vi "test Encode and Decoding Parameters for Payload.vi"() -> ()   [LabVIEW 2020, in "AIM ARINC 664 Scripting.lvclass"]
uses:
  AIM ARINC 664 Scripting.lvclass
  Shared/Encoding (Arinc664).ctl
  <vilib>/addons/_JKI Toolkits/VI Tester/TestCase.llb/TestCase.lvclass
  Engine/Implementation/Rx UDP Execution Unit/Rx UDP Execution Unit.lvclass
  C:/Program Files (x86)/National Instruments/LabVIEW 2020/vi.lib/addons/_JKI Toolkits/VI Tester/TestCase.llb/TestCase.lvclass
panel:
  out "Message Buffer out":u8[](array[numeric])
  out "Data":u8[](array[numeric])
  out "Array":dbl[](array[numeric])
  out "TestCase out":refnum<class "AIM ARINC 664 Scripting.lvclass">
  in  "TestCase in":refnum<class "AIM ARINC 664 Scripting.lvclass">
  out "error out":errorcluster
  in  "error in (no error)":errorcluster
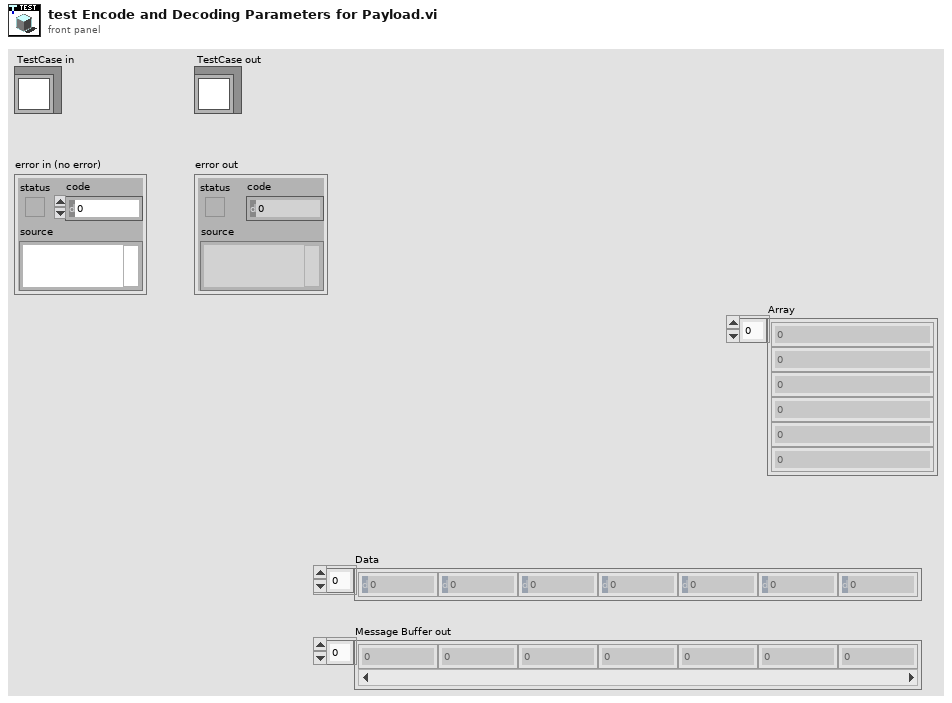
[diagram p1: front panel]
types:
  T1 = typedef "Encoding (Arinc664).ctl" = u16
  T2 = cluster{"start index":i32, "size":i32, "encoding":T1, "signed":bool, "scale multiplier":dbl, "scale offset":dbl}[]
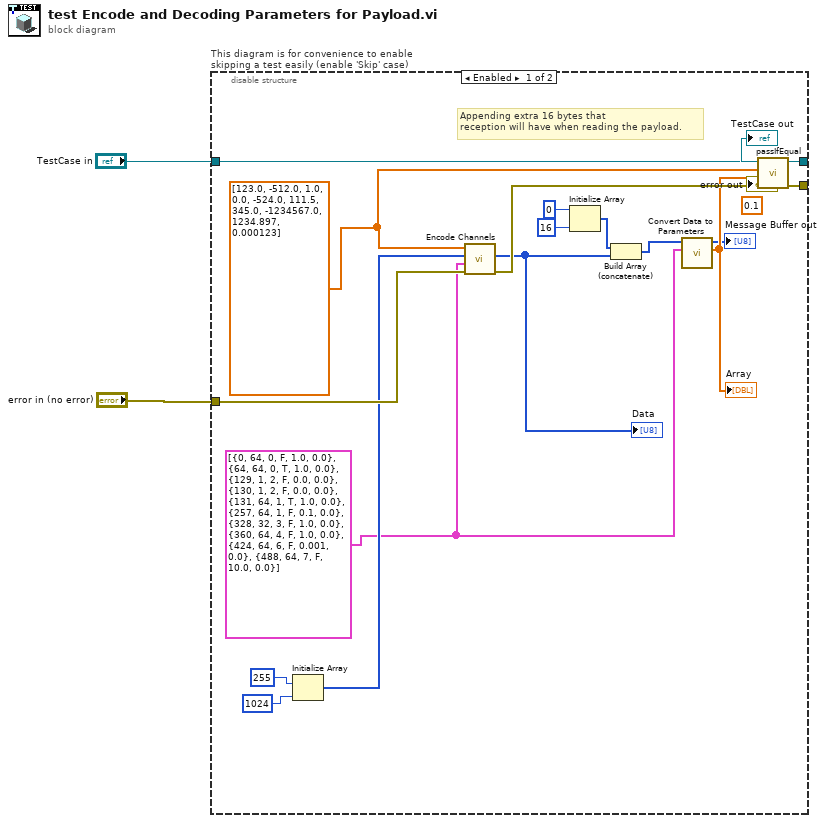
[diagram p0: block diagram]
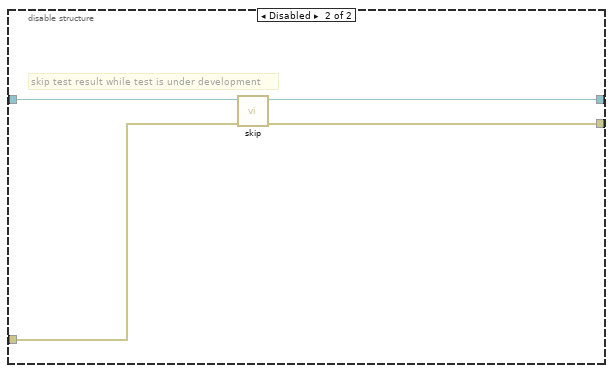
[diagram p2: hidden frame]
diagram:
  n1 = disable-structure "This diagram is for convenience to enable skipping a test easily (enable 'Skip' case)" shown="Enabled" {
    disable-tunnel: "TestCase in" -> [w16 w25]
    disable-tunnel: [w20 w23] -> w2
    disable-tunnel: [w21 w24] -> w3
    disable-tunnel: "error in (no error)" -> [w19 w22]
    frame Enabled {
      w5 = T2 [{"start index"=0, "size"=64, "encoding"=0, "signed"=FALSE, "scale multiplier"=1.0, "scale offset"=0.0}, {"start index"=64, "size"=64, "encoding"=0, "signed"=TRUE, "scale multiplier"=1.0, "scale offset"=0.0}, {"start index"=129, "size"=1, "encoding"=2, "signed"=FALSE, "scale multiplier"=0.0, "scale offset"=0.0}, {"start index"=130, "size"=1, "encoding"=2, "signed"=FALSE, "scale multiplier"=0.0, "scale offset"=0.0}, {"start index"=131, "size"=64, "encoding"=1, "signed"=TRUE, "scale multiplier"=1.0, "scale offset"=0.0}, {"start index"=257, "size"=64, "encoding"=1, "signed"=FALSE, "scale multiplier"=0.1, "scale offset"=0.0}, {"start index"=328, "size"=32, "encoding"=3, "signed"=FALSE, "scale multiplier"=1.0, "scale offset"=0.0}, {"start index"=360, "size"=64, "encoding"=4, "signed"=FALSE, "scale multiplier"=1.0, "scale offset"=0.0}, {"start index"=424, "size"=64, "encoding"=6, "signed"=FALSE, "scale multiplier"=0.001, "scale offset"=0.0}, {"start index"=488, "size"=64, "encoding"=7, "signed"=FALSE, "scale multiplier"=10.0, "scale offset"=0.0}] ("Parameters")
      w6 = dbl[] [123.0, -512.0, 1.0, 0.0, -524.0, 111.5, 345.0, -1234567.0, 1234.897, 0.000123] ("Values in")
      (unwired) 0.1 ("Value")
      # "Appending extra 16 bytes that \nreception will have when reading the payload."
      n2 = Initialize Array(255 ("dimension size"), 1024 ("dimension size")) -> (w7:i32[])
      n3 = call "Encode Channels.vi"("error in"=w19, "Parameters"=w5, "Data in"=w7, "Values in"=w6) -> ("error out"=w15:errorcluster, "Data out"=w8:u8[])  [unwired: 5 in, 1 out]
      "Data" <- w8
      n4 = Initialize Array(0 ("element"), 16 ("dimension size")) -> (w10:i32[])
      n5 = Build Array (concatenate)(w10, w8) -> (w9:i32[])
      n6 = call "Convert Data to Parameters.vi"("Parameters"=w5, "Message Buffer in"=w9) -> ("Array"=w14:dbl[], "Message Buffer out"=→"Message Buffer out":u8[])  [unwired: 8 in]
      "Array" <- w14
      n7 = call-dynamic "passIfEqual.vi"("error in (no error)"=w15, "y"=w14, "x"=w6, "TestCase in"=w16) -> ("error out"=w21:errorcluster, "TestCase out"=w20:refnum<class "AIM ARINC 664 Scripting.lvclass">)  [unwired: 6 in]
    }
    frame Disabled {
      # "skip test result while test is under development"
      n8 = call <vilib>:"skip.vi"("error in (no error)"=w22, "TestCase in"=w25) -> ("error out"=w24:errorcluster, "TestCase out"=w23:refnum<class "AIM ARINC 664 Scripting.lvclass">)  [unwired: 8 in]
    }
  }
  "error out" <- w3
  "TestCase out" <- w2
